vi "Update Item Overlay.vi"(8 "error in (no error)":errorcluster, 10 "Item":T1) -> (0 "error out":errorcluster)   [LabVIEW 2020, in "Icon Decorator V2.lvclass"]
doc: "Refresh the overlay for the Test Case class."
uses:
  Icon Decorator V2.lvclass
  <resource>/Framework/Providers/API/ItemRef.ctl
  <resource>/Framework/Providers/API/mxLvUpdateUI.ctl
  <resource>/Framework/Providers/API/mxLvOverlayState.ctl
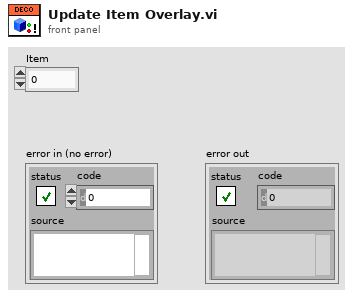
[diagram p1: front panel]
types:
  T1 = typedef "ItemRef.ctl" = u64
  T2 = typedef "mxLvUpdateUI.ctl" = cluster{"Action":u32, "Optional param 1":string, "Optional param 2":i32, "Optional param 3":string}
  T3 = typedef "mxLvOverlayState.ctl" = cluster{"Overlay Alias":string, "Active":bool}
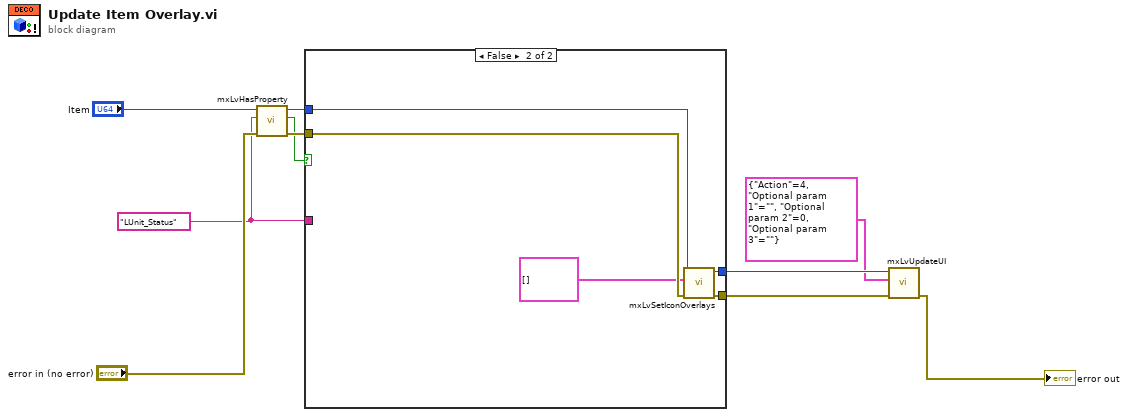
[diagram p0: block diagram]
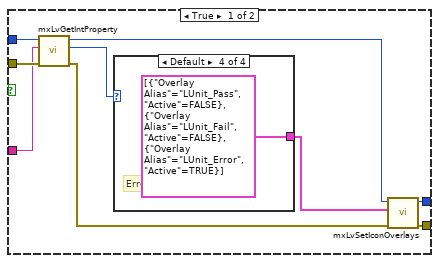
[diagram p2: hidden frame]
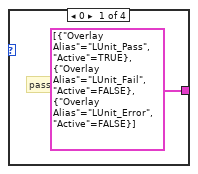
[diagram p3: hidden frame]
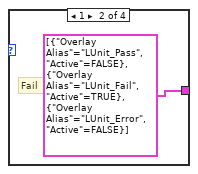
[diagram p4: hidden frame]
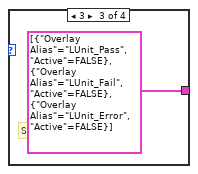
[diagram p5: hidden frame]
diagram:
  w5 = "LUnit_Status" ("Tag")
  n1 = call <resource>:"mxLvHasProperty.vi"("error in"="error in (no error)", "Tag"=w5, "Item"="Item") -> ("error out"=w7:errorcluster, "HasProperty"=w1:bool, "Item"=w8:T1)  [unwired: 6 in]
  n2 = case shown="False" w1 {
    tunnel: w8 -> [w19 w26]
    tunnel: w7 -> [w18 w25]
    tunnel: w5 -> [w17 _]
    tunnel: [w16 w28] -> w4
    tunnel: [w15 w27] -> w3
    frame True {
      n3 = call <resource>:"mxLvGetIntProperty.vi"("error in"=w18, "Tag"=w17, "Item"=w19) -> ("error out"=w12:errorcluster, "Value"=w11:i32, "Item"=w13:T1)  [unwired: 6 in]
      n4 = case shown="Default" w11 {
        tunnel: [T3[] [{"Overlay Alias"="LUnit_Pass", "Active"=TRUE}, {"Overlay Alias"="LUnit_Fail", "Active"=FALSE}, {"Overlay Alias"="LUnit_Error", "Active"=FALSE}] ("Array") T3[] [{"Overlay Alias"="LUnit_Pass", "Active"=FALSE}, {"Overlay Alias"="LUnit_Fail", "Active"=TRUE}, {"Overlay Alias"="LUnit_Error", "Active"=FALSE}] ("Array") T3[] [{"Overlay Alias"="LUnit_Pass", "Active"=FALSE}, {"Overlay Alias"="LUnit_Fail", "Active"=FALSE}, {"Overlay Alias"="LUnit_Error", "Active"=FALSE}] ("Array") T3[] [{"Overlay Alias"="LUnit_Pass", "Active"=FALSE}, {"Overlay Alias"="LUnit_Fail", "Active"=FALSE}, {"Overlay Alias"="LUnit_Error", "Active"=TRUE}] ("Array")] -> w14
        frame 0 {
          # "pass"
        }
        frame 1 {
          # "Fail"
        }
        frame 3 {
          # "Skip"
        }
        frame Default {
          # "Error"
        }
      }
      n5 = call <resource>:"mxLvSetIconOverlays.vi"("error in"=w12, "Overlay States"=w14, "Item"=w13) -> ("error out"=w16:errorcluster, "Item"=w15:T1)  [unwired: 7 in]
    }
    frame False {
      n6 = call <resource>:"mxLvSetIconOverlays.vi"("error in"=w25, "Overlay States"=T3[] [], "Item"=w26) -> ("error out"=w28:errorcluster, "Item"=w27:T1)  [unwired: 7 in]
    }
  }
  n7 = call <resource>:"mxLvUpdateUI.vi"("error in"=w4, "Update UI Settings"=T2 {"Action"=4, "Optional param 1"="", "Optional param 2"=0, "Optional param 3"=""}, "Item"=w3) -> ("error out"=→"error out":errorcluster)  [unwired: 7 in, 1 out]
